vi "Write Single Holding Register.vi"(8 "error in (no error)":errorcluster, 9 "holding register value":u16, 10 "address":u16, 11 "Modbus master in":refnum<class "Network Master.lvclass">) -> (0 "error out":errorcluster, 3 "Modbus master out":refnum<class "Network Master.lvclass">)   [LabVIEW 2021, in "Network Master.lvclass"]
doc: "Writes a value to a single holding register."
uses:
  Network Master.lvclass
  Modbus Data Unit/Modbus Data Unit.lvclass/Modbus Data Unit.ctl
  Network Master.lvclass/Network Master.ctl
  Modbus Data Unit/Construct PDU.vi
  Master Function Definition/Function code mismatch error.vi
  Data Model/Error Generator.vi
  Modbus Data Unit/Deconstruct PDU.vi
  Modbus Data Unit/Modbus Data Unit.lvclass
  Transmission Data Unit/Transmission Data Unit.lvclass
  Master Function Definition/Master Function Definition.lvclass
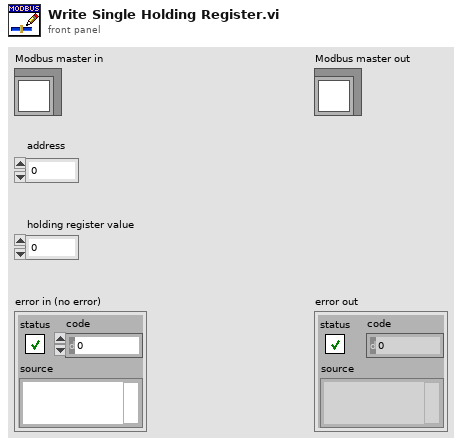
[diagram p1: front panel]
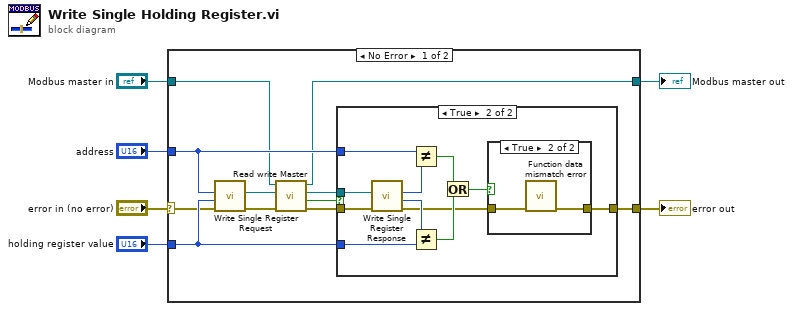
[diagram p0: block diagram]
diagram:
  n1 = case shown="No Error" "error in (no error)" {
    selector: "error in (no error)" -> [w7 w34]
    tunnel: "Modbus master in" -> [w8 w33]
    tunnel: [w9 w33] -> w4
    tunnel: [w16 w34] -> w3
    tunnel: "address" -> [w15 _]
    tunnel: "holding register value" -> [w14 _]
    frame No Error {
      n2 = call "Write Single Register Request.vi"("error in"=w7, "Register Value"=w14, "Starting Address"=w15) -> ("error out"=w17:errorcluster, "modbus data unit out"=w12:refnum<class "Modbus Data Unit.lvclass">)  [unwired: 7 in]
      n3 = call "Read write Master.vi"("error in (no error)"=w17, "Modbus data unit in"=w12, "Modbus master in"=w8) -> ("error out"=w13:errorcluster, "PDU valid?"=w11:bool, "Modbus data unit out"=w10:refnum<class "Modbus Data Unit.lvclass">, "Modbus master out"=w9:refnum<class "Network Master.lvclass">)  [unwired: 5 in]
      n4 = case shown="True" w11 {
        tunnel: [w18 w26] -> w16
        tunnel: w15 -> [_ w20]
        tunnel: w14 -> [_ w25]
        tunnel: w13 -> [w18 w23]
        tunnel: w10 -> [_ w22]
        frame False {
        }
        frame True {
          n5 = call "Write Single Register Response.vi"("error in"=w23, "modbus data unit in"=w22) -> ("error out"=w21:errorcluster, "Number of Coils"=w24:u16, "Address"=w19:u16)  [unwired: 7 in]
          n6 = Not Equal?(x=w20, y=w19) -> (x != y?=w28:bool)
          n7 = Not Equal?(x=w24, y=w25) -> (x != y?=w29:bool)
          n8 = Or(x=w28, y=w29) -> (x .or. y?=w27:bool)
          n9 = case shown="True" w27 {
            tunnel: [w30 w32] -> w26
            tunnel: w21 -> [w30 w31]
            frame False {
            }
            frame True {
              n10 = call "Function data mismatch error.vi"("error in (no error)"=w31) -> ("error out"=w32:errorcluster)  [unwired: 10 in]
            }
          }
        }
      }
    }
    frame Error {
    }
  }
  "error out" <- w3
  "Modbus master out" <- w4
